vi "VISA(Create).vi"(8 "error in (no error)":errorcluster caption="错误输入（无错误）") -> (0 "error out":errorcluster caption="错误输出", 2 "F?":bool, 3 "VISA resource name out":refnum<visa-resource-name>)   [LabVIEW 2020, in "人体健康监测系统.lvclass"]
uses:
  <vilib>/Instr/_visa.llb/VISA Configure Serial Port (Instr).vi
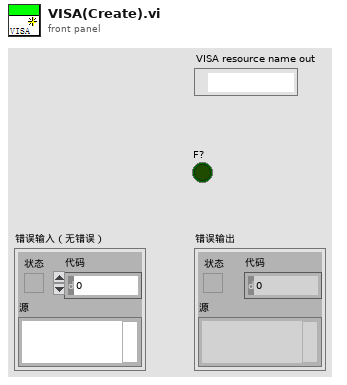
[diagram p1: front panel]
types:
  T1 = typedef "人体健康监测系统.lvclass/串口配置.ctl" = cluster{"COM":refnum<visa-resource-name>, "baud rate (9600)":u32, "data bits (8)":u16, "parity (0:none)":enum16{"None", "Odd", "Even", "Mark", "Space"}, "stop bits (10: 1 bit)":u16}
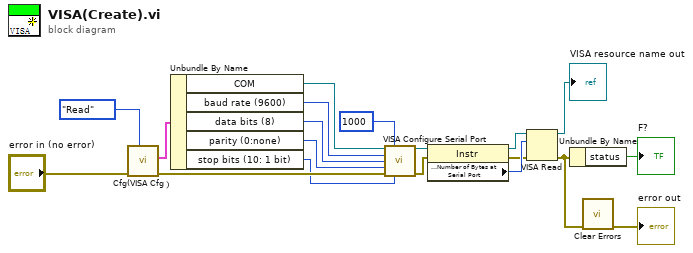
[diagram p0: block diagram]
diagram:
  n1 = call "Cfg(VISA Cfg）.vi"("R/W"=enum16{"Read", "Write"}."Read", "error in (no error)"="error in (no error)") -> ("error out"=w14:errorcluster, "串口配置"=w13:T1)  [unwired: 8 in]
  n2 = Unbundle By Name(w13) -> ("COM"=w12:refnum<visa-resource-name>, "baud rate (9600)"=w11:u32, "data bits (8)"=w10:u16, "parity (0:none)"=w9:enum16{"None", "Odd", "Even", "Mark", "Space"}, "stop bits (10: 1 bit)"=w8:u16)
  n3 = call-poly "VISA Configure Serial Port"("VISA resource name"=w12, "timeout (10sec)"=u32 1000, "baud rate (9600)"=w11, "data bits (8)"=w10, "parity (0:none)"=w9, "error in (no error)"=w14, "stop bits (10: 1 bit)"=w8) -> ("VISA resource name out"=w6:refnum<visa-resource-name>, "error out"=w5:errorcluster)  [unwired: 7 in]
  n4 = property class="Instr"(reference=w6, error in=w5) -> (reference out=w4:refnum<visa-resource-name>, error out=w2:errorcluster, "Serial Settings:Number of Bytes at Serial Port"=w3:u32)
  n5 = VISA Read(VISA resource name=w4, byte count=w3, error in (no error)=w2) -> (VISA resource name out=→"VISA resource name out":refnum<visa-resource-name>, error out=w1:errorcluster)  [unwired: 2 out]
  n6 = Unbundle By Name(w1) -> ("status"=→"F?":bool)
  n7 = call <vilib>:"Clear Errors.vi"("error in (no error)"=w1) -> ("error out"=→"error out":errorcluster)  [unwired: 5 in, 1 out]
